vi "Pre Launch Init.vi"(11 "Vehicle Position Interface Simulation in":refnum<class "Vehicle Position Interface Simulation.lvclass">) -> (0 "error out":errorcluster, 3 "Vehicle Position Interface Simulation out":refnum<class "Vehicle Position Interface Simulation.lvclass">)   [LabVIEW 2012, in "Vehical Position Interface Simulation.lvlib" / "Vehicle Position Interface Simulation.lvclass"]
doc: "(<B>Filename</B>: Actor Framework.lvlib:Actor.lvclass:Pre Launch Init.vi)\n\nDefines behavior that occurs after the Launch Actor method is invoked but before the actor's Actor Core method begins running.\n\nThe Pre Launch Init method is guaranteed to finish before the Launch Actor method returns to its caller and before the actor itself receives any messages. Any references that the Pre Launch Init method obtains are guaranteed to have the same lifetime as the actor itself. Any errors that the Pre Launch Init method returns will abort the launch.\n\nBy default, this method does nothing. A descendant class may override it to define behavior."
uses:
  Vehicle Position Interface Simulation.lvclass
  Vehical Position Interface API/Vehical Position Interface API/Vehicle Position Interface API.lvclass
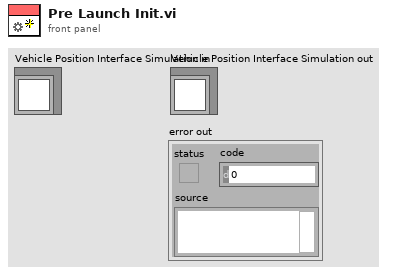
[diagram p1: front panel]
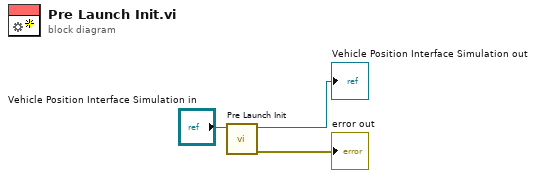
[diagram p0: block diagram]
diagram:
  n1 = call-parent "Pre Launch Init.vi"("Actor in"="Vehicle Position Interface Simulation in") -> ("error out"=→"error out":errorcluster, "Actor out"=→"Vehicle Position Interface Simulation out":refnum<class "Vehicle Position Interface Simulation.lvclass">)  [unwired: 9 in]
